vi "Acceleration Conversion Module.vi"(6 "Array Input (1 row 6 col)":u8[][](array[numeric]), 8 "Second column":i32, 9 "First column":i32) -> (3 "Acceleration [g] -2.0<->+2.0":dbl)   [LabVIEW 2025]
panel:
  # "Outputs"
  # "Inputs"
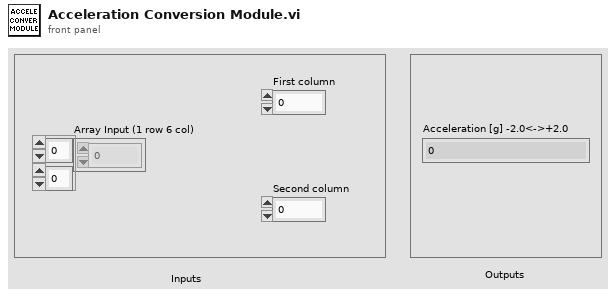
[diagram p1: front panel]
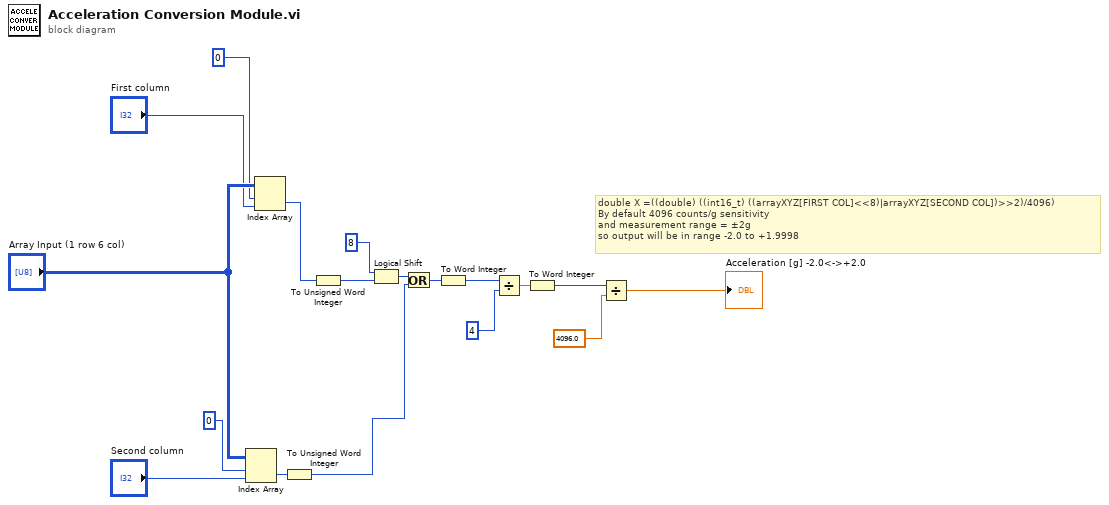
[diagram p0: block diagram]
diagram:
  # "double X =((double) ((int16_t) ((arrayXYZ[FIRST COL]<<8)|arrayXYZ[SECOND COL])>>2)/4096)\nBy default 4096 counts/g sensitivity\nand measurement range = ±2g\nso output will be in range -2.0 to +1.9998"
  n1 = Index Array(array="Array Input (1 row 6 col)", index (row)=0, index (col)="Second column") -> (element=w14:u8)
  n2 = Index Array(array="Array Input (1 row 6 col)", index (row)=0, index (col)="First column") -> (element=w8:u8)
  n3 = To Unsigned Word Integer(number=w14) -> (unsigned 16bit integer=w15:u16)
  n4 = To Unsigned Word Integer(number=w8) -> (unsigned 16bit integer=w7:u16)
  n5 = Logical Shift(y=u16 8, x=w7) -> (x << y=w11:u16)
  n6 = Or(x=w11, y=w15) -> (x .or. y?=w13:u16)
  n7 = To Word Integer(number=w13) -> (16bit integer=w18:i16)
  n8 = Divide(x=w18, y=i16 4) -> (x/y=w16:dbl)
  n9 = To Word Integer(number=w16) -> (16bit integer=w12:i16)
  n10 = Divide(x=w12, y=4096.0) -> (x/y=→"Acceleration [g] -2.0<->+2.0":dbl)
